vi "Pulse_Length.vi"(11 "Trigger":bool[](array[boolean])) -> (1 "Rising Index":i32[](array[numeric]), 2 "Mean Pulse Length":dbl, 3 "Histogram Graph":T1)   [LabVIEW 2012]
uses:
  <vilib>/Analysis/baseanly.llb/Mean (DBL).vi
  <vilib>/Analysis/NI_AALPro.lvlib
  <vilib>/Analysis/NI_AALBase.lvlib
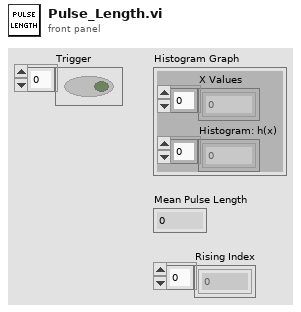
[diagram p1: front panel]
types:
  T1 = cluster{"X Values":dbl[], "Histogram: h(x)":i32[]}
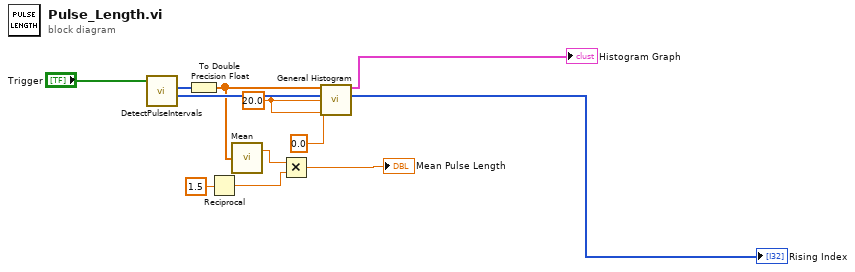
[diagram p0: block diagram]
diagram:
  w4 = 20.0 ("max")
  n1 = call "DetectPulseIntervals.vi"("Binary array probe"="Trigger") -> ("Rising Index"=→"Rising Index":i32[], "Pulse lenghts out"=w10:i32[])  [unwired: 6 in, 3 out]
  n2 = To Double Precision Float(number=w10) -> (double precision float=w9:dbl[])
  n3 = Reciprocal(x=1.5) -> (1/x=w8:dbl)
  n4 = call-poly <vilib>:"Mean.vi"("X"=w9) -> ("mean"=w7:dbl)  [unwired: 1 out]
  n5 = Multiply(x=w7, y=w8) -> (x*y=→"Mean Pulse Length":dbl)
  n6 = call <vilib>:"General Histogram.vi"("X"=w9, "max"=w4, "min"=0.0, "# bins"=w4) -> ("Histogram Graph"=→"Histogram Graph":T1)  [unwired: 7 in, 4 out]
